vi "Port Under Mouse.vi"(8 "error in (no error)":errorcluster, 10 "point":cluster{"x":i16, "y":i16}, 11 "FSM in":refnum<class "FSM.Graph.lvclass">) -> (0 "error out":errorcluster, 1 "found?":bool, 2 "Port":refnum<class "FSM.Port.lvclass">, 3 "FSM out":refnum<class "FSM.Graph.lvclass">)   [LabVIEW 2015, in "FSM.Graph.lvclass"]
uses:
  FSM.Graph.lvclass
  FSM.Port/FSM.Port.lvclass
  FSM.Graph.lvclass/FSM.Graph.ctl
  FSM.Node/FSM.Node.lvclass
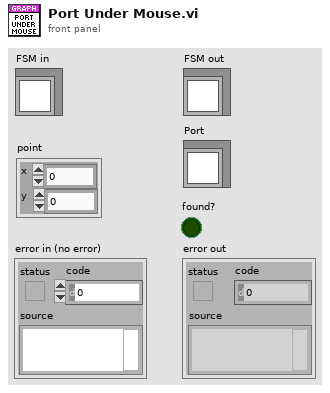
[diagram p1: front panel]
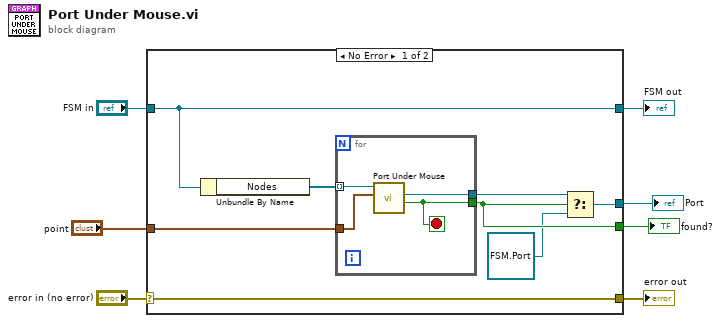
[diagram p0: block diagram]
diagram:
  n1 = case shown="No Error" "error in (no error)" {
    selector: "error in (no error)" -> [w15 w21]
    tunnel: [w15 w21] -> w6
    tunnel: [w14 w20] -> w4
    tunnel: "FSM in" -> [w14 w20]
    tunnel: "point" -> [w12 _]
    tunnel: [w9 _] -> w2
    tunnel: [w10 _] -> w1
    frame No Error {
      n2 = Unbundle By Name(w14) -> ("Nodes"=w13:refnum<class "FSM.Node.lvclass">[])
      n3 = for {
        tunnel: w13 -> [w19] mode=indexing
        tunnel: w12 -> [w18]
        tunnel: [w17] -> w10
        tunnel: [w16] -> w11
        stop <- w17 stop-if-true
        n4 = call "Port Under Mouse.vi"("point"=w18, "FSM in"=w19) -> ("found?"=w17:bool, "Port"=w16:refnum<class "FSM.Port.lvclass">)  [unwired: 6 in, 2 out]
      }
      n5 = Select(t=w11, s=w10, f=refnum<class "FSM.Port.lvclass"> refnum) -> (s? t:f=w9:refnum<class "FSM.Port.lvclass">)
    }
    frame Error {
    }
  }
  "error out" <- w6
  "FSM out" <- w4
  "Port" <- w2
  "found?" <- w1
